vi "SL2_AD_DLL_Phoibos_GetDeviceState.vi"(0 "dll_path":path, 1 "pHandle_in":u32, 2 "dev_type":T1, 3 "error in":errorcluster) -> (5 "path out":path, 7 "state":T2 items=["Off"=-1, "Standby"=0, "On"=1], 8 "error out":errorcluster)   [LabVIEW 2020]
uses:
  DEFINITIONS/DEF_dev_state.ctl
  DEFINITIONS/DEF_dev_type.ctl
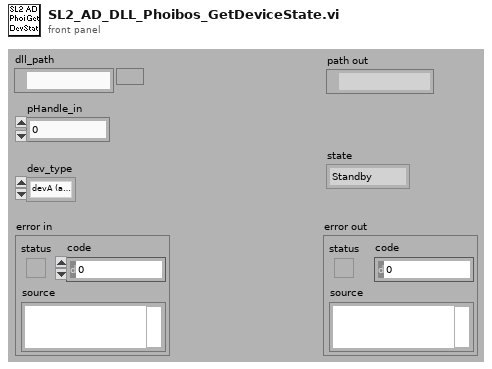
[diagram p1: front panel]
types:
  T1 = typedef "DEF_dev_type.ctl" = enum32{"devA (analyzer)", "devD (detector)"}
  T2 = typedef "DEF_dev_state.ctl" = i32
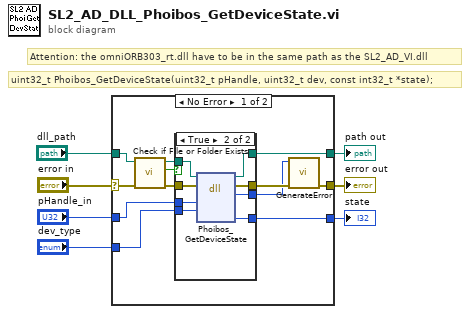
[diagram p0: block diagram]
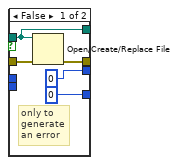
[diagram p2: hidden frame]
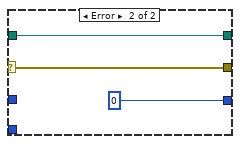
[diagram p3: hidden frame]
diagram:
  # "uint32_t Phoibos_GetDeviceState(uint32_t pHandle, uint32_t dev, const int32_t *state);"
  # "Attention: the omniORB303_rt.dll have to be in the same path as the SL2_AD_VI.dll"
  n1 = case shown="No Error" "error in" {
    selector: "error in" -> [w17 w35]
    tunnel: "dev_type" -> [w19 _]
    tunnel: [w12 w35] -> w6
    tunnel: [w18 w34] -> w5
    tunnel: "dll_path" -> [w16 w34]
    tunnel: "pHandle_in" -> [w15 _]
    tunnel: [w14 0 ("state")] -> w1
    frame No Error {
      n2 = call <vilib>:"Check if File or Folder Exists.vi"("error in (no error)"=w17, "path"=w16) -> ("error out"=w10:errorcluster, "file or folder exists?"=w8:bool, "dup path"=w9:path)  [unwired: 7 in]
      n3 = case shown="True" w8 {
        tunnel: w19 -> [_ w31]
        tunnel: [w24 w28] -> w13
        tunnel: [w22 w26] -> w18
        tunnel: [u32 0 ("error_code") w30] -> w11
        tunnel: w10 -> [w23 w32]
        tunnel: w9 -> [w22 w27]
        tunnel: w15 -> [_ w29]
        tunnel: [0 ("pHandle") w25] -> w14
        frame False {
          # "only to generate an error"
          n4 = Open/Create/Replace File(file path (use dialog)=w22, error in=w23) -> (error out=w24:errorcluster)  [unwired: 4 in, 2 out]
        }
        frame True {
          n5 = dll-call lib="C:/Programme/SPECS/SpecsLab2/programming/LabView7.1/SL2_AD_VI.dll" fn="Phoibos_GetDeviceState"(path in=w27, error in=w32, "pHandle"=w29, "dev"=w31) -> (path out=w26:path, error out=w28:errorcluster, "error_code"=w30:u32, "state"=w25:i32)  [unwired: 4 in]
        }
      }
      n6 = call "GenerateError.vi"("error in"=w13, "error_code"=w11) -> ("error out"=w12:errorcluster)  [unwired: 9 in]
    }
    frame Error {
    }
  }
  "state" <- w1
  "error out" <- w6
  "path out" <- w5
